vi "Display Update Timer FGV.vi"(2 "Times of Sample Rate":u32) -> (0 "Update Control Data?":bool=TRUE)   [LabVIEW 2018]
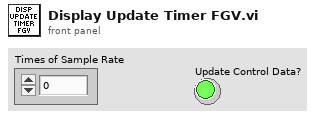
[diagram p1: front panel]
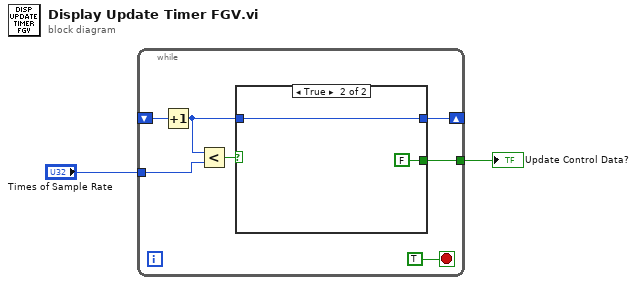
[diagram p0: block diagram]
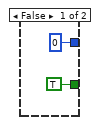
[diagram p2: hidden frame]
diagram:
  n1 = while {
    shift-right: [w7] -> _
    shift-left: _ -> [w5]
    tunnel: [w6] -> w2
    tunnel: "Times of Sample Rate" -> [w3]
    stop <- TRUE stop-if-true
    n2 = Increment(x=w5) -> (x+1=w4:u8)
    n3 = Less?(x=w4, y=w3) -> (x < y?=w8:bool)
    n4 = case shown="True" w8 {
      tunnel: w4 -> [_ w12]
      tunnel: [u8 0 w12] -> w7
      tunnel: [TRUE FALSE] -> w6
      frame False {
      }
      frame True {
      }
    }
  }
  "Update Control Data?" <- w2
